vi "instrumentProperties_gainLevels_available.vi"(0 "reference":refnum<class "OSA300.lvclass">, 5 "error in (no error)":errorcluster) -> (10 "status FTSLib":string, 14 "duplicate reference":refnum<class "OSA300.lvclass">, 16 "gainLevels at sensitivity":dbl[](array[numeric]), 19 "error out":errorcluster)   [LabVIEW 2010, in "OSA300.lvclass"]
doc: "Resolution depends on resolution mode."
uses:
  OSA300.lvclass
  _dll/LVLib/FTSLib.lvlib
  _OSAchannel_class/OSAchannel.lvclass
  OSA.lvclass
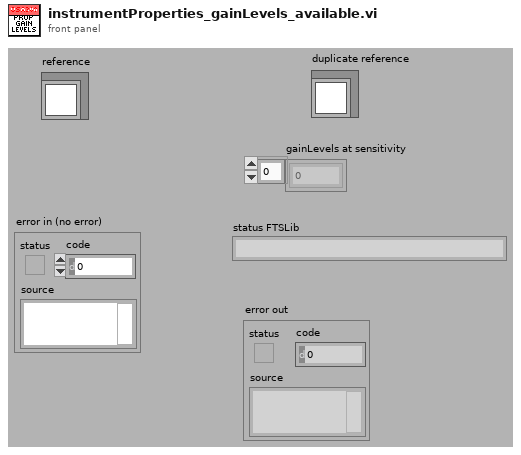
[diagram p1: front panel]
types:
  T1 = typedef "OSA20X_misc.lvlib/amplifier_sort.ctl" = enum16{"amp_unknown", "amp_se_8", "amp_se_12_lg", "amp_se_12", "amp_se_16", "amp_diff_8", "amp_diff_12_lg", "amp_diff_12_ir", "amp_diff_16", "amp_other", "amp_other_2"}
  T2 = typedef "OSA20X_misc.lvlib/detector_sort.ctl" = enum16{"unknown", "Silicon", "Silicon PIN", "Silicon MPPC", "InGaAs", "InGaAs ext low", "InGaAs ext high", "InAs", "InAsSb", "InSb", "MCT", "other", "other2", "other3"}
  T3 = typedef "OSA20X_misc.lvlib/interferogram_smoothing.ctl" = enum16{"NONE", "BINOMIAL", "SAVITSKY_GOLAY", "FOURIER", "MOVING_AVERAGE", "GAUSSIAN"}
  T4 = typedef "OSA20X_misc.lvlib/PDTemperatureMode.ctl" = enum16{"cool: better sensitivity/noise floor", "warm: extended wl range"}
  T5 = cluster{"waveMin (cm-1)":sgl, "waveMax (cm-1)":sgl, "gainOffset_auto":bool, "gain":i32, "gain levels nr":u16, "offset":i32, "offset max":u16, "damper available":bool, "damper active":bool, "amplifier sort":T1, "detector sort":T2, "channelIdx global":u16, "spectrIdx":u16, "waveMeter on":bool, "ref gainLevels rel.":refnum<data-value>, "intfgrm_smooth_width":u16, "intfgrm_smooth_nrOfPasses":u16, "intfgrm_smooth":T3, "adc #bits":u16, "temp Variable":bool, "spectr_smooth":T3, "spectr_smooth_width":u16, "spectr_smooth_nrOfPasses":u16, "PD sensitivity mode":T4, "damper auto":bool}
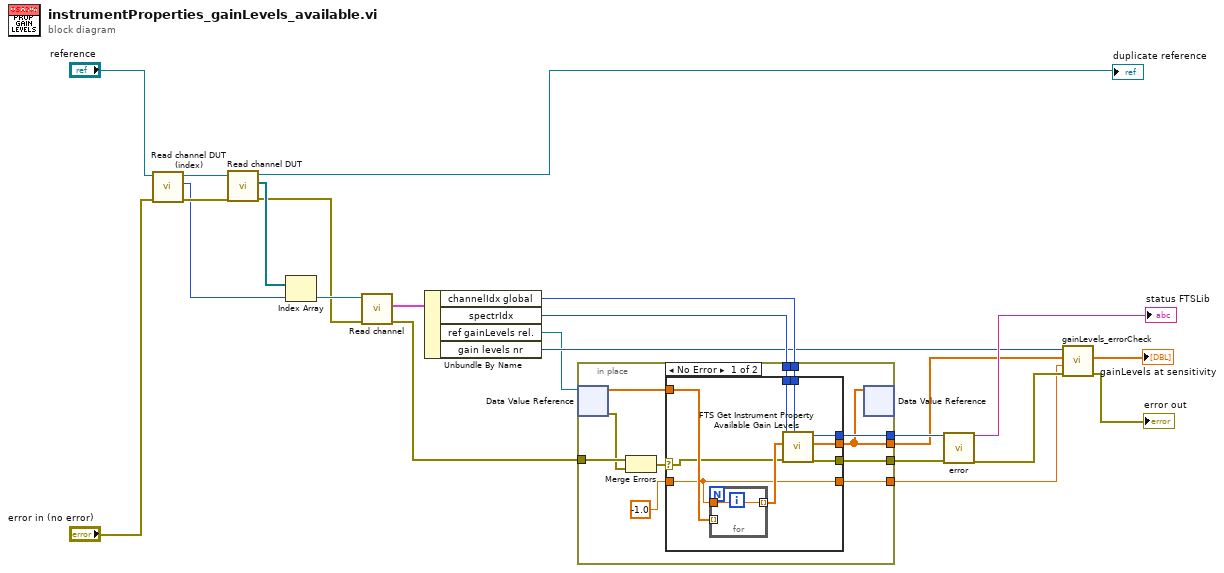
[diagram p0: block diagram]
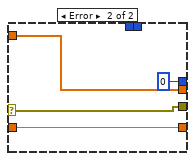
[diagram p2: hidden frame]
diagram:
  n1 = call "Read channel DUT (index).vi"("error in (no error)"="error in (no error)", "OSA300 in"="reference") -> ("error out"=w20:errorcluster, "channel ifrgrm (index)"=w17:i32, "OSA300 out"=w19:refnum<class "OSA300.lvclass">)  [unwired: 7 in]
  n2 = call "Read channel DUT.vi"("error in (no error)"=w20, "OSA300 in"=w19) -> ("error out"=w10:errorcluster, "channel DUT"=w18:refnum<class "OSAchannel.lvclass">[], "OSA300 out"=→"duplicate reference":refnum<class "OSA300.lvclass">)  [unwired: 7 in]
  n3 = Index Array(array=w18, index=w17) -> (element=w11:refnum<class "OSAchannel.lvclass">)
  n4 = call "Read channel.vi"("error in (no error)"=w10, "OSAchannel in"=w11) -> ("error out"=w9:errorcluster, "channel"=w21:T5)  [unwired: 7 in, 1 out]
  n5 = Unbundle By Name(w21) -> ("channelIdx global"=w22:u16, "spectrIdx"=w23:u16, "ref gainLevels rel."=w1:refnum<data-value>, "gain levels nr"=w5:u16)
  n6 = in-place {
    in-place-border: w23 -> [w34]
    in-place-border: w22 -> [w33]
    in-place-border: [w32] -> w16
    in-place-border: [w31] -> w15
    in-place-border: w9 -> [w28]
    in-place-border: [w25] -> w6
    in-place-border: [w30] -> w4
    n7 = in-place-dvr #1(w1) -> (w29:dbl[], w27:errorcluster)
    n8 = Merge Errors(w28, w27) -> (w26:errorcluster)
    n9 = case shown="No Error" w26 {
      selector: w26 -> [w36 w46]
      tunnel: w34 -> [w43 _]
      tunnel: w33 -> [w42 _]
      tunnel: [w41 w46] -> w32
      tunnel: [w40 u32 0 ("function return")] -> w31
      tunnel: [w38 w48] -> w25
      tunnel: [w35 w45] -> w30
      tunnel: w29 -> [w37 w48]
      tunnel: -1.0 -> [w35 w45]
      frame No Error {
        n10 = for {
          tunnel: w35 -> [w44]
          tunnel: [w44] -> w39 mode=indexing
          tunnel: w37 -> [_] mode=indexing
        }
        n11 = call "FTS Get Instrument Property Available Gain Levels.vi"("channel"=w42, "error in (no error)"=w36, "GainLevels"=w39, "specIndex"=w43) -> ("error out"=w41:errorcluster, "GainLevels out"=w38:dbl[], "function return"=w40:u32)  [unwired: 5 in]
      }
      frame Error {
      }
    }
    n12 = in-place-dvr #1(w25) -> ()  [unwired: 2 out]
  }
  n13 = call "error.vi"("result code"=w15, "error in (no error)"=w16) -> ("status"=→"status FTSLib":string, "error out"=w7:errorcluster)  [unwired: 15 in, 1 out]
  n14 = call "gainLevels_errorCheck.vi"("error in"=w7, "search value"=w4, "GainLevel array"=w6, "gain levels nr max"=w5) -> ("error out"=→"error out":errorcluster, "gain levels active"=→"gainLevels at sensitivity":dbl[])  [unwired: 6 in]
